vi "CreateMessageName.vi"(8 "error in (no error)":errorcluster, 11 "Message in":T1) -> (0 "error out":errorcluster, 3 "Message out":T1)   [LabVIEW 2017, in "MessageGen.lvlib"]
uses:
  <vilib>/addons/InsightCM/MessageBus/CodeGen/MessageGen.lvlib
  <vilib>/addons/InsightCM/MessageBus/CodeGen/controls/MessageData.ctl
  <vilib>/addons/InsightCM/MessageBus/CodeGen/controls/MessageType.ctl
  <vilib>/addons/InsightCM/MessageBus/CodeGen/controls/Parameter.ctl
  <vilib>/addons/InsightCM/MessageBus/CodeGen/controls/ParameterType.ctl
  <vilib>/LabVIEW Icon API/API_Text.ctl
  <vilib>/LabVIEW Icon API/LabVIEW Icon API.lvlib
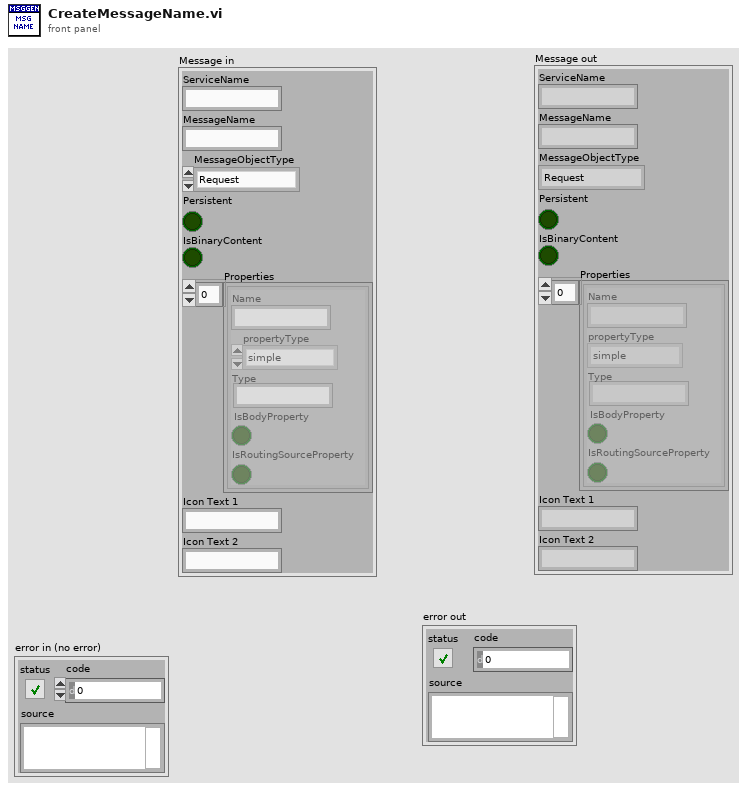
[diagram p1: front panel]
types:
  T1 = typedef "MessageGen.lvlib/MessageData.ctl" = cluster{"ServiceName":string, "MessageName":string, "MessageObjectType":T2, "Persistent":bool, "IsBinaryContent":bool, "Properties":T3[], "Icon Text 1":string, "Icon Text 2":string}
  T2 = typedef "MessageGen.lvlib/MessageType.ctl" = enum16{"Request", "Response", "Broadcast", "RoutedMessage"}
  T3 = typedef "MessageGen.lvlib/Parameter.ctl" = cluster{"Name":string, "propertyType":T4, "Type":string, "IsBodyProperty":bool, "IsRoutingSourceProperty":bool}
  T4 = typedef "MessageGen.lvlib/ParameterType.ctl" = enum16{"simple", "bytearray", "dateTime", "list", "map", "object"}
  T5 = typedef "LabVIEW Icon API.lvlib/API_Text.ctl" = cluster{"Line 1 text":string, "Line 2 text":string, "Line 3 text":string, "Line 4 text":string}
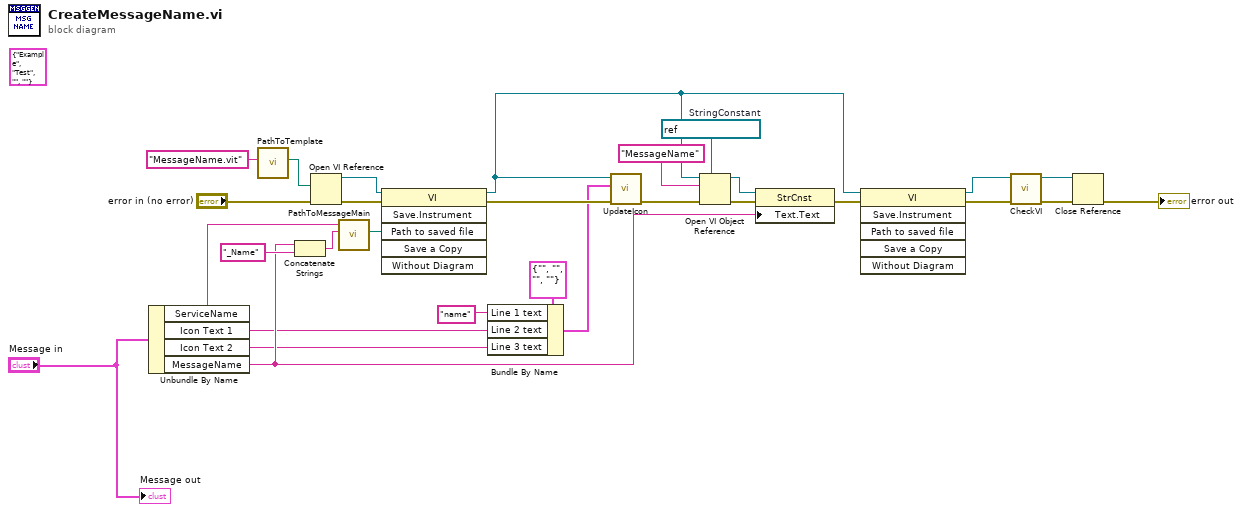
[diagram p0: block diagram]
diagram:
  (unwired) T5 {"Line 1 text"="Example", "Line 2 text"="Test", "Line 3 text"="", "Line 4 text"=""} ("Text")
  w25 = refnum<vi> refnum  # StringConstant
  n1 = Unbundle By Name("Message in") -> ("ServiceName"=w18:string, "Icon Text 1"=w3:string, "Icon Text 2"=w2:string, "MessageName"=w13:string)
  n2 = call <vilib>:"PathToTemplate.vi"("TemplateName"="MessageName.vit") -> ("Path"=w27:path)  [unwired: 10 in]
  n3 = Concatenate Strings(w13, "_Name" ("string")) -> (w20:string)
  n4 = Open VI Reference(vi path=w27, error in (no error)="error in (no error)") -> (vi reference=w23:refnum<vi>, error out=w22:errorcluster)  [unwired: 4 in]
  n5 = call <vilib>:"PathToMessageMain.vi"("VIName"=w20, "Service"=w18) -> ("Path"=w17:path)  [unwired: 9 in]
  n6 = invoke class="VI" method="Save.Instrument"(reference=w23, error in=w22, "Path to saved file"=w17) -> (reference out=w7:refnum<vi>, error out=w28:errorcluster)  [unwired: 3 in, 4 out]
  n7 = Bundle By Name(cluster=T5 {"Line 1 text"="", "Line 2 text"="", "Line 3 text"="", "Line 4 text"=""} ("Text"), "Line 1 text"="name" ("method"), "Line 2 text"=w3, "Line 3 text"=w2) -> (w1:T5)
  n8 = call <vilib>:"UpdateIcon.vi"("error in (no error)"=w28, "Text"=w1, "VI Refnum in"=w7) -> ("error out"=w29:errorcluster)  [unwired: 7 in, 1 out]
  n9 = Open VI Object Reference(7:w25, 8:w29, 10:"MessageName" ("name/order"), 11:w7) -> (0:w15:errorcluster, 3:w14:refnum<vi>)
  n10 = property class="StrCnst"(reference=w14, error in=w15, "Text.Text"=w13) -> (error out=w6:errorcluster)  [unwired: 1 out]
  n11 = invoke class="VI" method="Save.Instrument"(reference=w7, error in=w6) -> (reference out=w9:refnum<vi>, error out=w11:errorcluster)  [unwired: 4 in, 4 out]
  n12 = call <vilib>:"CheckVI.vi"("error in (no error)"=w11, "VI ref"=w9) -> ("error out"=w12:errorcluster, "VI ref out"=w10:refnum<vi>)  [unwired: 8 in]
  n13 = Close Reference(reference=w10, error in (no error)=w12) -> (error out=→"error out":errorcluster)
  "Message out" <- "Message in"
